vi "Task Generation V.vi"(11 "Generation Channels":tag="cDAQ9188XT-1947DFEMod5/ao0") -> (0 "error out":errorcluster, 3 "Refnum out":refnum<k21>)   [LabVIEW 2018]
uses:
  <vilib>/DAQmx/create/channels.llb/DAQmx Create Channel (AO-Voltage-Basic).vi
  <vilib>/DAQmx/configure/timing.llb/DAQmx Timing (Sample Clock).vi
  Samples per channle (Generation) - Global Variable.vi
panel:
  in  "fs - rate":dbl=1000.0 format="%#_13g"
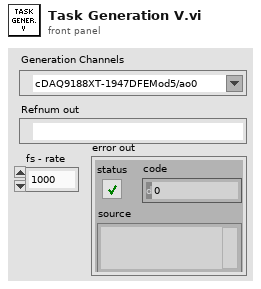
[diagram p1: front panel]
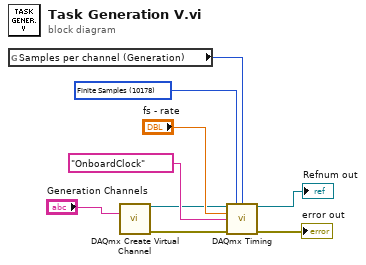
[diagram p0: block diagram]
diagram:
  w6 = 10178 items=["Finite Samples"=10178, "Continuous Samples"=10123, "Hardware Timed Single Point"=12522] ("sample mode")
  n1 = global read "Samples per channle (Generation) - Global Variable.vi" "Samples per channel (Generation)"() -> (w1:i32)
  n2 = call-poly <vilib>:"DAQmx Create Virtual Channel.vi"("physical channels"="Generation Channels") -> ("task out"=w3:refnum<k21>, "error out"=w4:errorcluster)  [unwired: 13 in]
  n3 = call-poly <vilib>:"DAQmx Timing.vi"("task/channels in"=w3, "sample mode"=w6, "samples per channel"=w1, "rate"="fs - rate", "source"=tag "OnboardClock", "error in"=w4) -> ("task out"=→"Refnum out":refnum<k21>, "error out"=→"error out":errorcluster)  [unwired: 8 in]
